vi "CheckIfStringArraysAreEqual-1D.vi"(10 "Array2":string[](array[string]), 11 "Array1":string[](array[string])) -> (3 "Equal?":bool)   [LabVIEW 2018]
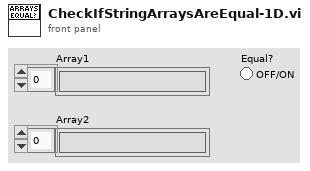
[diagram p1: front panel]
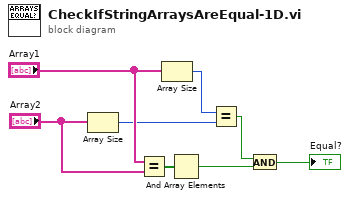
[diagram p0: block diagram]
diagram:
  n1 = Array Size(array="Array2") -> (size(s)=w2:i32)
  n2 = Equal?(x="Array1", y="Array2") -> (x = y?=w1:bool[])
  n3 = Array Size(array="Array1") -> (size(s)=w3:i32)
  n4 = And Array Elements(Boolean array=w1) -> (logical AND=w5:bool)
  n5 = Equal?(x=w3, y=w2) -> (x = y?=w4:bool)
  n6 = And(x=w4, y=w5) -> (x .and. y?=→"Equal?":bool)
